vi "Process.vi"(8 "error in":errorcluster, 11 "Instrument":refnum<class "Instrument.lvclass">) -> (0 "error out":errorcluster, 3 "Instrument out":refnum<class "Instrument.lvclass">)   [LabVIEW 2016, in "Instrument.lvclass"]
doc: "---------------------------------------------------------------\nJKI State Machine Objects™\nhttp://jki.net/state-machine-objects/\nCopyright (C) 2005-2015, JKI <info@jki.net>\nALL RIGHTS RESERVED"
uses:
  Instrument.lvclass
  <vilib>/JKI/JKI SMO/SMO/SMO.lvclass
  <vilib>/JKI/JKI SMO/SMO/Typedefs/Parent Call--Enum.ctl
  levylab_util_remote/src/RemoteControl/RemoteControl.lvclass
  levylab_util_remote/src/RemoteControl/Typedefs/PublicEvents--RemoteControl.ProcessCommand.ctl
  levylab_util_remote/src/RemoteControl/Typedefs/PrivateEvents--RemoteControl.CommandResponse.ctl
  C:/Program Files (x86)/National Instruments/LabVIEW 2016/vi.lib/JKI/JKI SMO/SMO/SMO.lvclass
panel:
  out "ProcessCommand.Data":string
  out "ProcessCommand.Command":string
  # "INSTRUMENT"
  # "Receives command from Remote process"
  # "For instructions on how to use the JKI State Machine Objects, examples and video tutorials, visit:\nhttp://jki.net/state-machine-objects/\n\nJKI State Machine Objects™\nhttp://jki.net/state-machine-objects/\nCopyright (C) 2005-2015, JKI <info@jki.net>\nALL RIGHTS RESERVED"
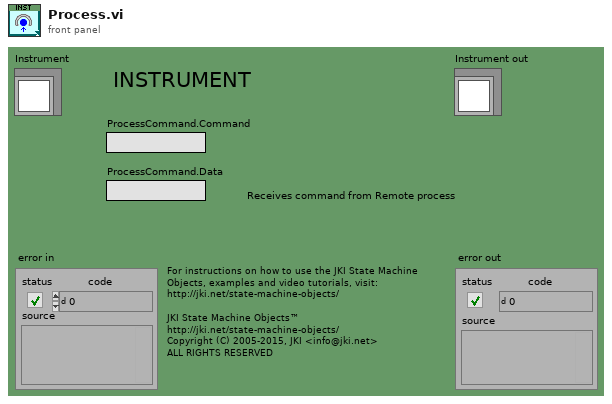
[diagram p1: front panel]
types:
  T1 = typedef "SMO.lvclass/Parent Call--Enum.ctl" = enum16{"Allows parent to run", "Does not request parent to run"}
  T2 = enum32{"invalid app kind", "Development System", "Run Time System", "Student Edition", "Embedded LabVIEW", "Evaluation", "Custom"}
  T3 = enum32{"Invalid", "Standard", "Closed", "Hidden", "Minimized", "Maximized"}
  T4 = enum32{"Bad", "Idle", "Run top level", "Running"}
  T5 = typedef "RemoteControl.lvclass/PrivateEvents--RemoteControl.CommandResponse.ctl" = cluster{"Command Reply":string, "Data Reply":string}
  T6 = typedef "RemoteControl.lvclass/PublicEvents--RemoteControl.ProcessCommand.ctl" = cluster{"Command":string, "Data":string}
  T7 = cluster{"Core":cluster{"Current VI Reference":refnum<vi>, "Close Panel on Exit?":bool, "error":errorcluster}, "Self Reference":refnum<class "Instrument.lvclass">, "Your string data":string, "RemoteControl out":refnum<class "RemoteControl.lvclass">, "ProcessCommand":T6}
  T8 = typedef "Instrument.lvclass/PrivateEvents--Instrument.SetPort.ctl" = i32
  T9 = typedef "Instrument.lvclass/PrivateEvents--Instrument.SetCommands.ctl" = string[]
  T10 = typedef "Instrument.lvclass/PrivateEvents--Instrument.SetAllowedRemote.ctl" = string
  T11 = cluster{"Current VI Reference":refnum<vi>, "Close Panel on Exit?":bool, "error":errorcluster}
  T12 = typedef "SMO.lvclass/Protected Events.ctl" = cluster{"StopProcesses":refnum<user-event>, "AbortProcesses":refnum<user-event>, "Config Changed":refnum<user-event>, "Dependency":refnum<user-event>}
  T13 = typedef "RemoteControl.lvclass/PublicEvents--Cluster.ctl" = cluster{"ProcessCommand":refnum<user-event>}
  T14 = typedef "Instrument.lvclass/PrivateEvents--Cluster.ctl" = cluster{"SetPort":refnum<user-event>, "SetCommands":refnum<user-event>, "SetAllowedRemote":refnum<user-event>}
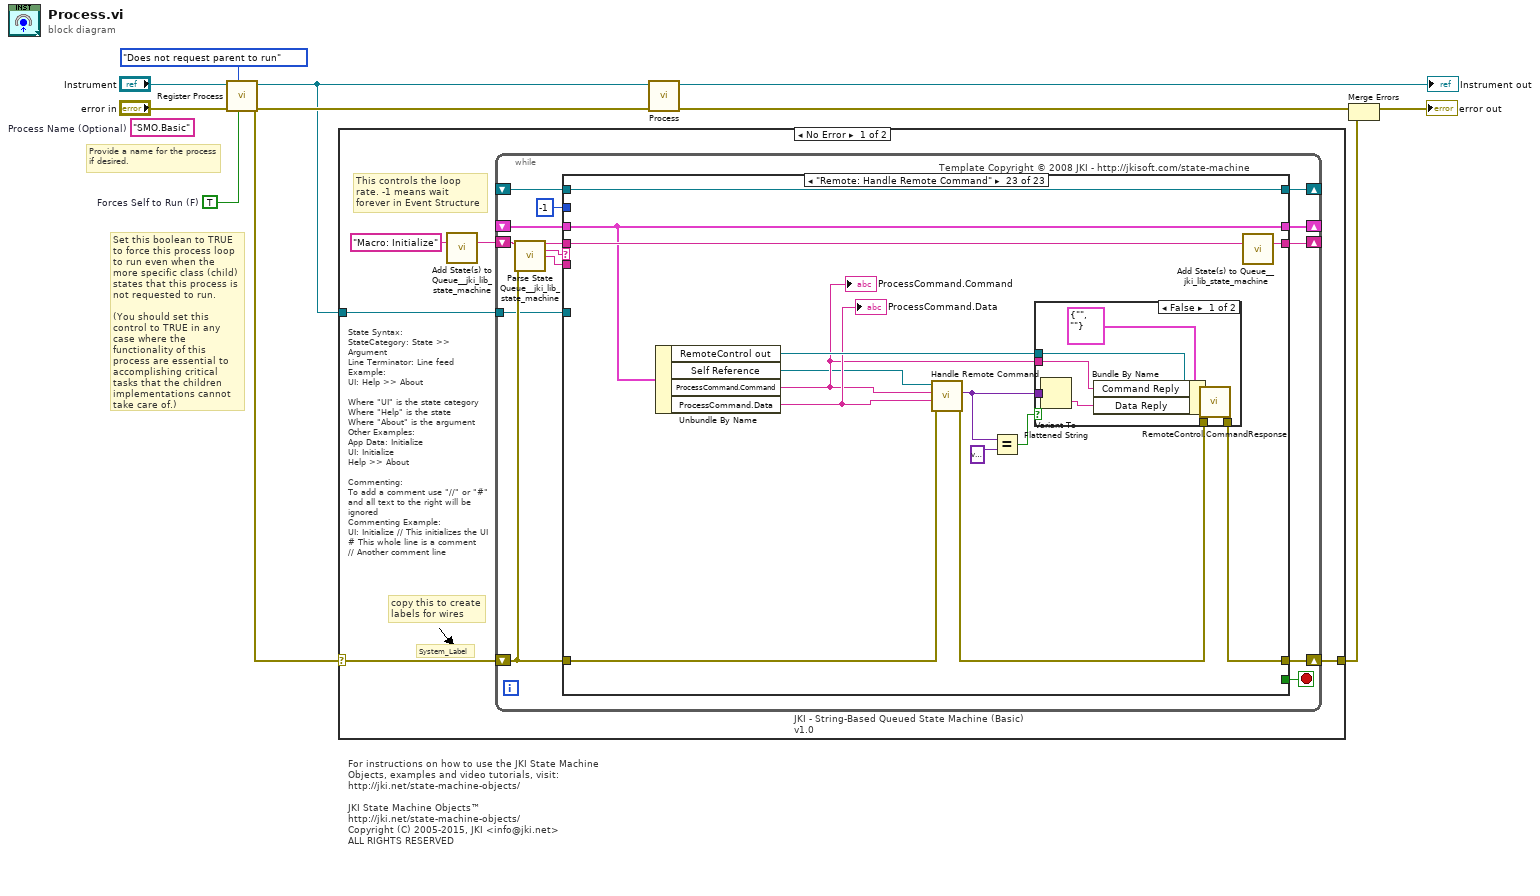
[diagram p0: block diagram]
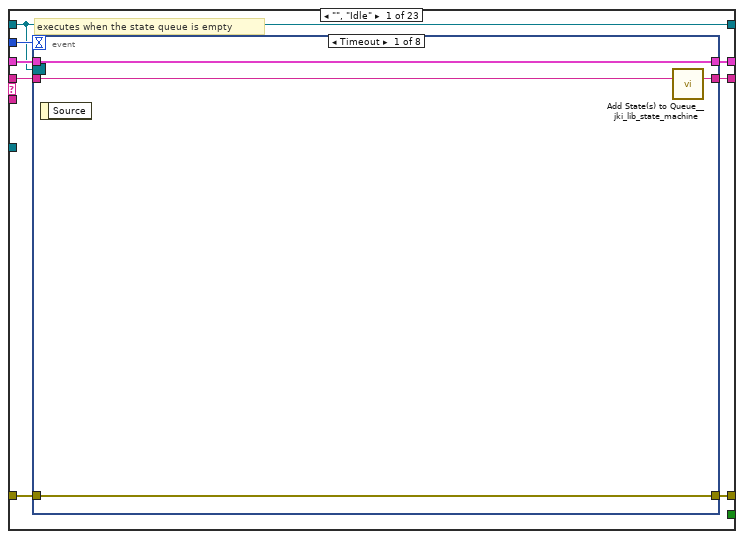
[diagram p2: hidden frame]
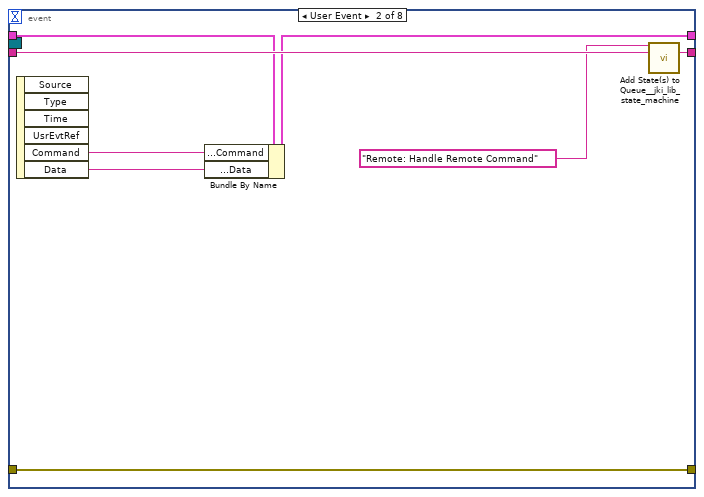
[diagram p3: hidden frame]
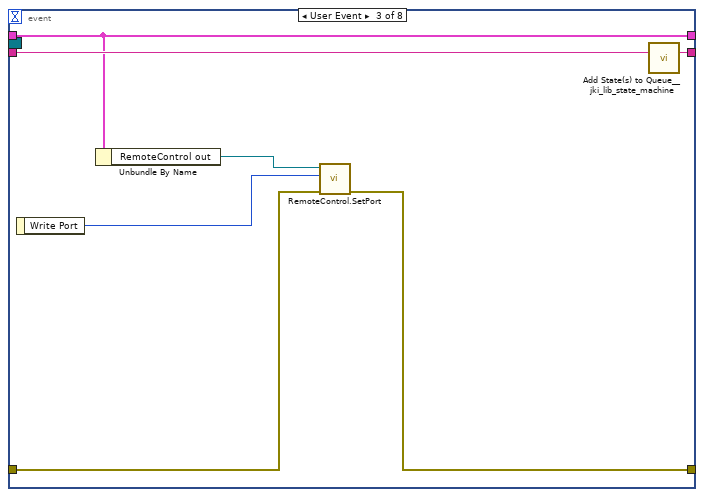
[diagram p4: hidden frame]
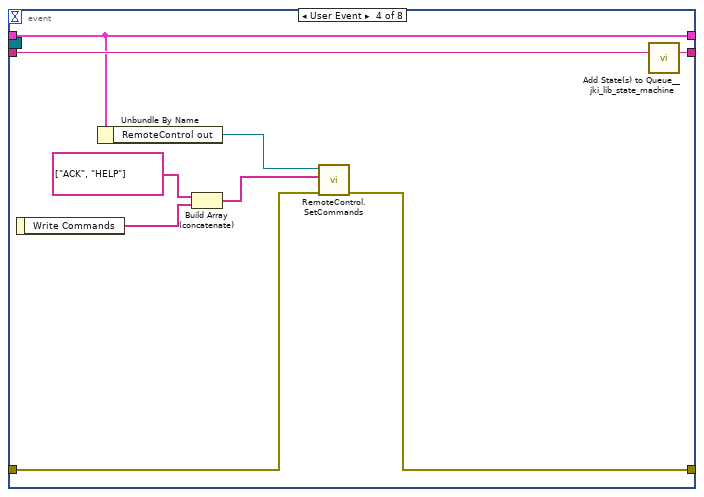
[diagram p5: hidden frame]
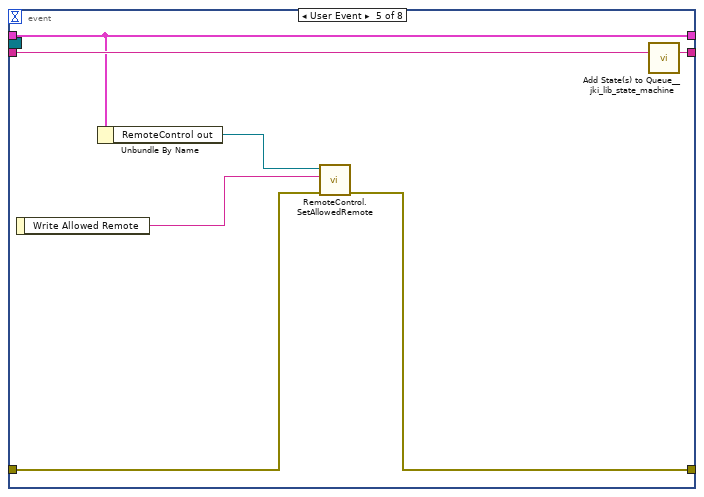
[diagram p6: hidden frame]
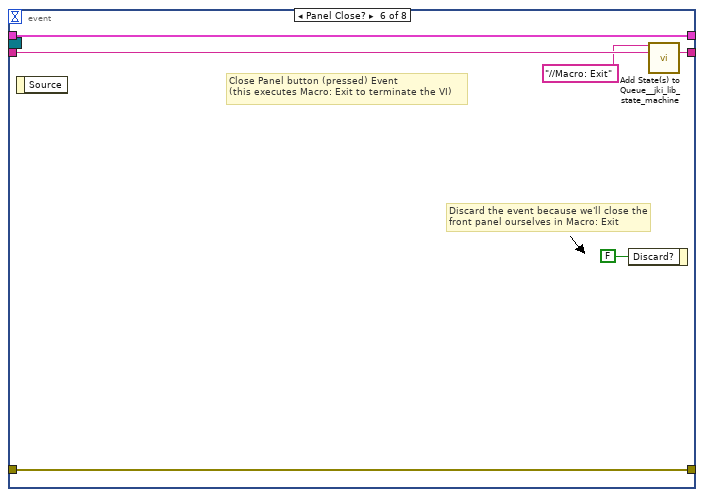
[diagram p7: hidden frame]
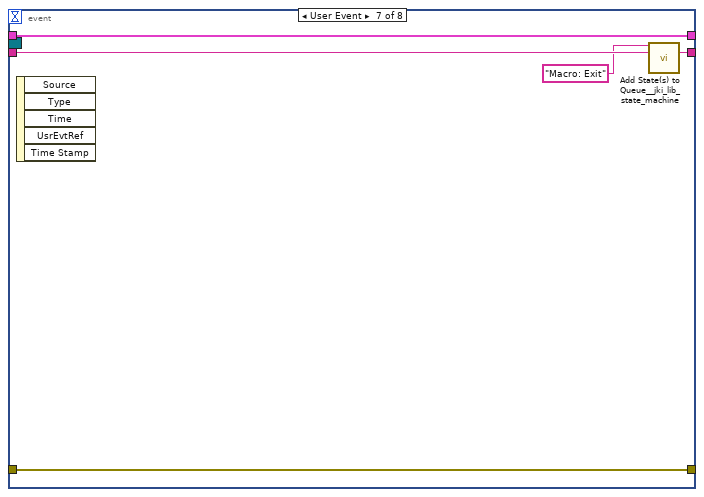
[diagram p8: hidden frame]
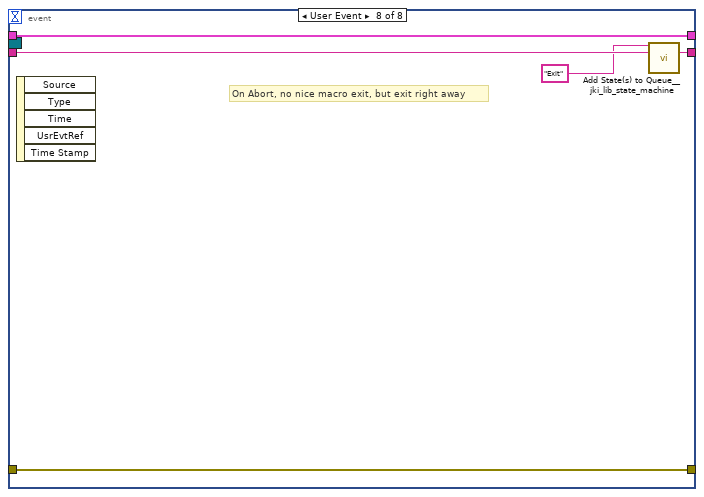
[diagram p9: hidden frame]
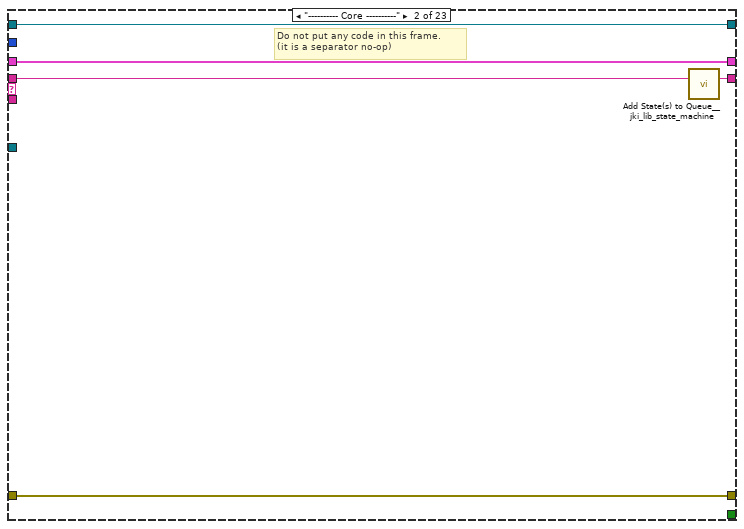
[diagram p10: hidden frame]
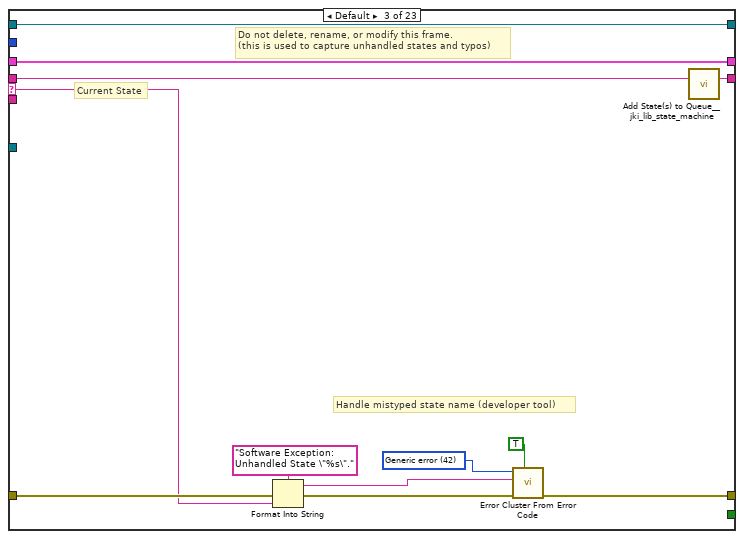
[diagram p11: hidden frame]
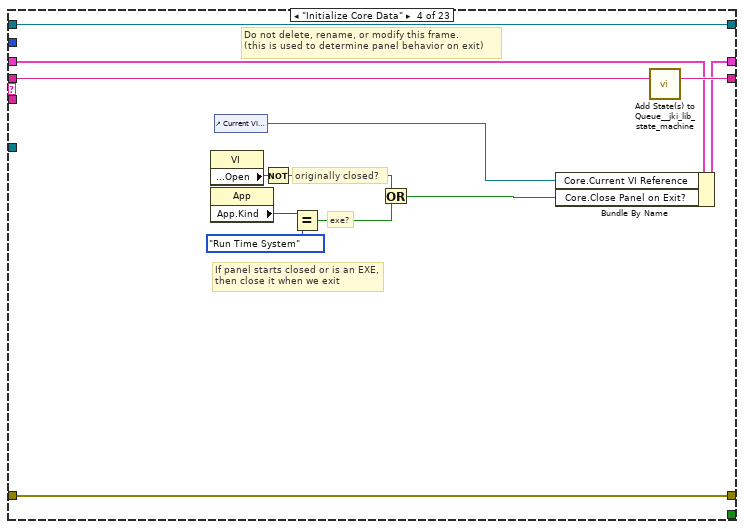
[diagram p12: hidden frame]
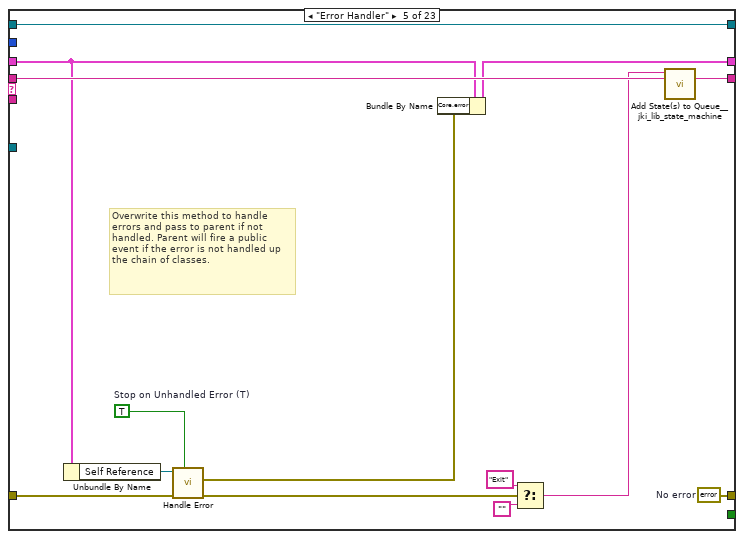
[diagram p13: hidden frame]
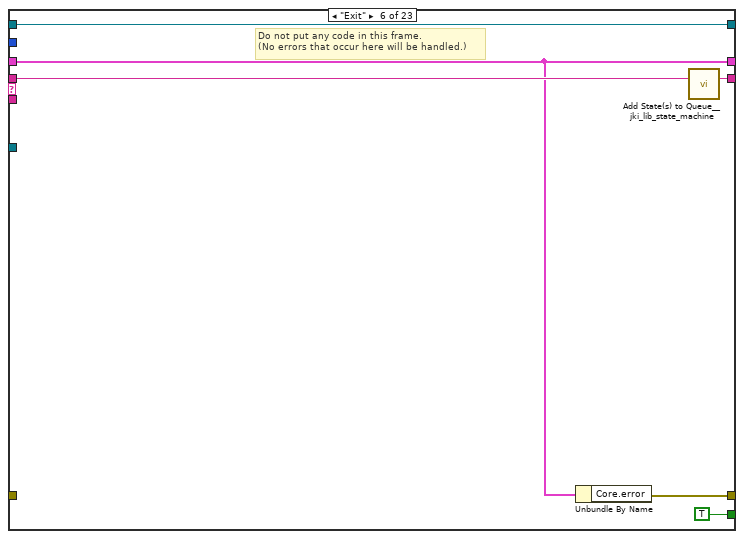
[diagram p14: hidden frame]
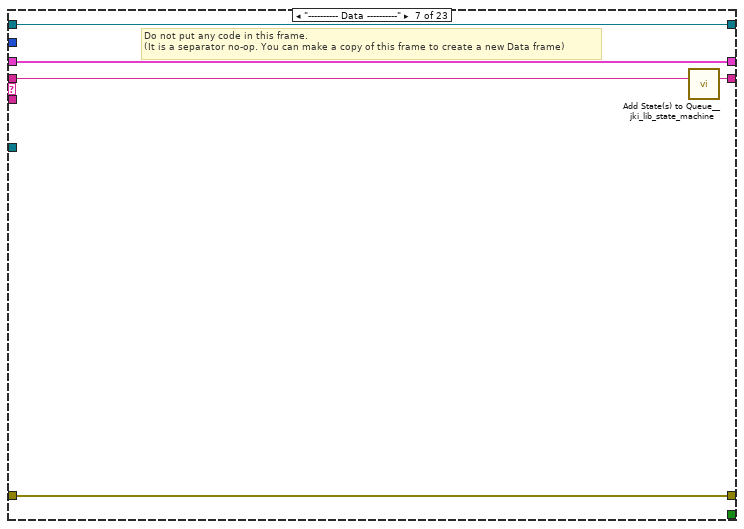
[diagram p15: hidden frame]
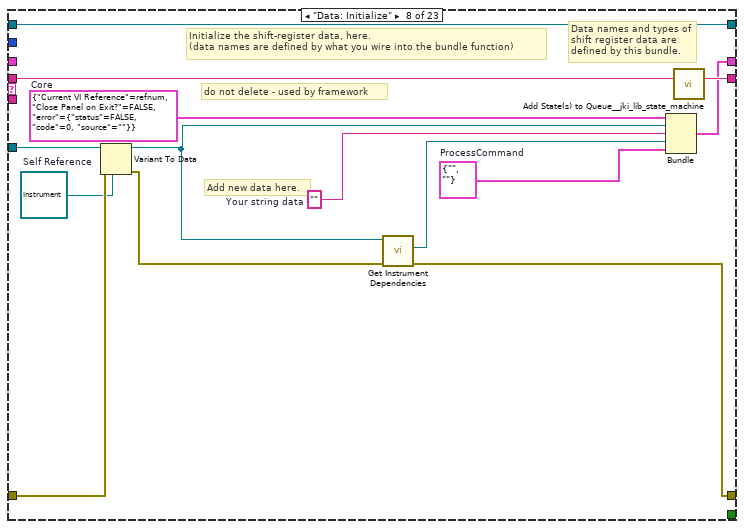
[diagram p16: hidden frame]
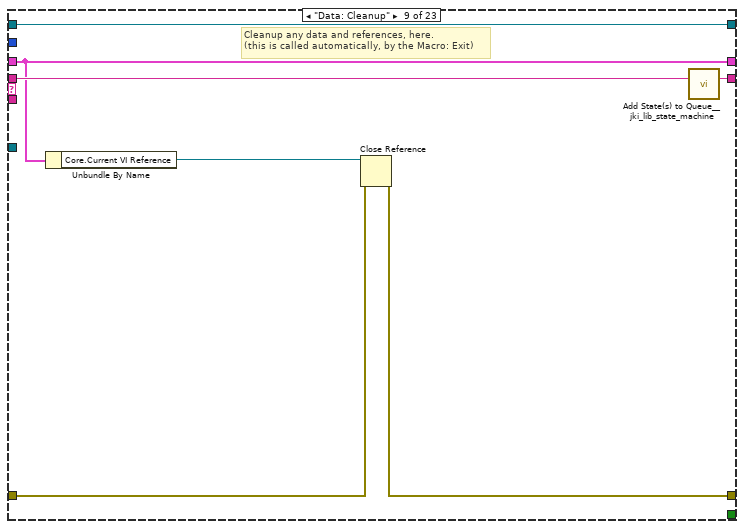
[diagram p17: hidden frame]
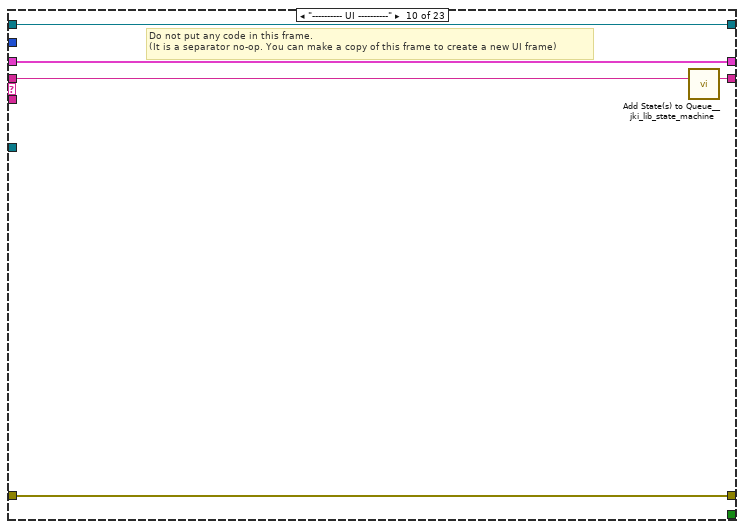
[diagram p18: hidden frame]
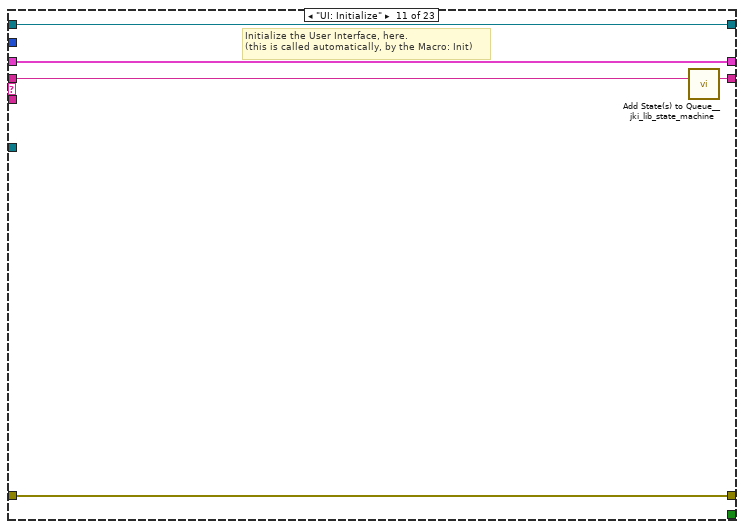
[diagram p19: hidden frame]
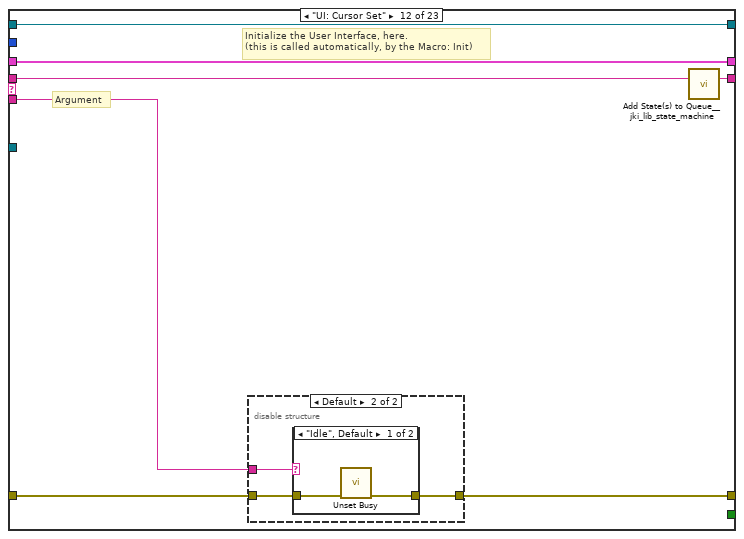
[diagram p20: hidden frame]
diagram:
  w1 = TRUE  # Forces Self to Run (F)
  (unwired) "SMO.Basic"  # Process Name (Optional)
  # "Provide a name for the process\nif desired."
  # "Set this boolean to TRUE to force this process loop to run even when the more specific class (child) states that this process is not requested to run.\n\n(You should set this control to TRUE in any case where the functionality of this process are essential to accomplishing critical tasks that the children implementations cannot take care of.)"
  # "For instructions on how to use the JKI State Machine Objects, examples and video tutorials, visit:\nhttp://jki.net/state-machine-objects/\n\nJKI State Machine Objects™\nhttp://jki.net/state-machine-objects/\nCopyright (C) 2005-2015, JKI <info@jki.net>\nALL RIGHTS RESERVED"
  n1 = call <vilib>:"Register Process.vi"("Forces Self to Run (F)"=w1, "Parent Call"=Parent_Call--Enum."Does not request parent to run", "error in (no error)"="error in", "SMO"="Instrument") -> ("error out"=w7:errorcluster, "SMO out"=w6:refnum<class "Instrument.lvclass">)  [unwired: 6 in]
  n2 = case shown="No Error" w7 {
    selector: w7 -> [w12 w329]
    tunnel: w6 -> [w13 _]
    tunnel: [w11 w329] -> w3
    frame No Error {
      # "State Syntax:\nStateCategory: State >> Argument\nLine Terminator: Line feed\nExample:\nUI: Help >> About\n\nWhere \"UI\" is the state category\nWhere \"Help\" is the state\nWhere \"About\" is the argument\nOther Examples:\nApp Data: Initialize\nUI: Initialize\nHelp >> About\n\nCommenting:\nTo add a comment use \"//\" or \"#\" and all text to the right will be ignored\nCommenting Example:\nUI: Initialize // This initializes the UI\n# This whole line is a comment\n// Another comment line"
      # "copy this to create labels for wires"
      # "This controls the loop rate. -1 means wait forever in Event Structure"
      # "System_Label"
      n3 = call <vilib>:"Add State(s) to Queue__jki_lib_state_machine.vi"("State(s) in (\"\")"="Macro: Initialize") -> ("States Out"=w15:string)  [unwired: 14 in]
      n4 = while "JKI - String-Based Queued State Machine (Basic) v1.0" {
        shift-right: [w22] -> _
        shift-left: _ -> [w21]
        shift-right: [w25] -> w11
        shift-left: w12 -> [w19]
        shift-right: [w24] -> _
        shift-left: w15 -> [w26]
        tunnel: w13 -> [w18]
        shift-right: [w17] -> _
        shift-left: _ -> [w16]
        stop <- w23 stop-if-true
        # "Template Copyright © 2008 JKI - http://jkisoft.com/state-machine"
        n5 = call <vilib>:"Parse State Queue__jki_lib_state_machine.vi"("State Queue"=w26, "Error In (no error)"=w19) -> ("Remaining States"=w28:string, "Current State"=w29:string, "Arguments"=w27:string)  [unwired: 11 in]
        n6 = case shown="\"Remote: Handle Remote Command\"" w29 {
          selector: w29 -> [_ _ w95 _ _ _ _ _ _ _ _ _ _ _ _ _ _ _ _ _ _ _ _]
          tunnel: w28 -> [w37 w93 w99 w118 w132 w138 w143 w157 w164 w169 w174 w181 w197 w229 w243 w257 w262 w273 w278 w294 w300 w305 w319]
          tunnel: w27 -> [_ _ _ _ _ _ _ _ _ _ _ w175 w191 _ _ _ _ _ _ _ _ _ _]
          tunnel: w21 -> [w35 w90 w97 w109 w126 w134 w140 _ w159 w166 w172 w179 w193 w226 w239 w248 w259 w270 w275 w292 w298 w303 w309]
          tunnel: [w34 w91 w101 w115 w127 w133 w141 w146 w160 w167 w171 w176 w194 w227 w241 w255 w260 w264 w276 w288 w296 w301 w310] -> w25
          tunnel: w19 -> [w33 w91 w100 w115 w128 _ w141 w153 w161 w167 w171 w177 w195 w227 w241 w255 w260 w265 w276 w284 w296 w301 w312]
          tunnel: [w36 w92 w98 w117 w131 w137 w142 w156 w163 w168 w173 w180 w196 w228 w242 w256 w261 w272 w277 w293 w299 w304 w318] -> w24
          tunnel: [_ _ _ _ _ TRUE _ _ _ _ _ _ _ _ _ _ _ _ _ _ _ _ _] -> w23
          tunnel: [w32 w90 w97 w116 w125 w134 w140 w155 w159 w166 w172 w179 w193 w226 w239 w248 w259 w270 w275 w292 w298 w303 w309] -> w22
          tunnel: -1 ("Timeout") -> [w31 _ _ _ _ _ _ _ _ _ _ _ _ _ _ _ _ _ _ _ _ _ _]
          tunnel: w18 -> [_ _ _ _ _ _ _ w151 _ _ _ _ _ _ _ _ _ _ _ _ _ _ _]
          tunnel: [w30 w89 w94 w106 w130 w135 w139 w150 w158 w165 w170 w178 w190 w225 w240 w249 w258 w271 w274 w291 w297 w302 w317] -> w17
          tunnel: w16 -> [w30 w89 w94 w106 w130 w135 w139 w150 w158 w165 w170 w178 w190 w225 w240 w249 w258 w271 w274 _ w297 w302 w317]
          frame "", "Idle" {
            # "executes when the state queue is empty"
            n7 = event shown="[0] Timeout" {
              selector: w30 -> [_ _ _ _ _ _ _ _]
              dyn-events: _ -> [_ _ _ _ _ _ _ _]
              timeout: w31 -> [_ _ _ _ _ _ _ _]
              tunnel: w37 -> [w41 w49 w56 w65 w72 w78 w83 w88]
              tunnel: [w40 w48 w55 w64 w71 w77 w82 w87] -> w36
              tunnel: w35 -> [w39 w46 w54 w63 w70 w75 w80 w85]
              tunnel: [w38 w47 w51 w61 w67 w76 w81 w86] -> w34
              tunnel: w33 -> [w38 w47 w52 w62 w68 w76 w81 w86]
              tunnel: [w39 w45 w54 w63 w70 w75 w80 w85] -> w32
              event Timeout {
                n8 = event-data() -> ()  [unwired: 1 in, 1 out]
                n9 = call <vilib>:"Add State(s) to Queue__jki_lib_state_machine.vi"("State(s) in (\"\")"=w41) -> ("States Out"=w40:string)  [unwired: 14 in]
              }
              event User Event {
                n10 = event-data() -> ("Command"=w44:string, "Data"=w43:string)  [unwired: 1 in, 4 out]
                n11 = Bundle By Name(cluster=w46, "ProcessCommand.Command"=w44, "ProcessCommand.Data"=w43) -> (w45:T7)
                n12 = call <vilib>:"Add State(s) to Queue__jki_lib_state_machine.vi"("State(s) in Front (\"\")"="Remote: Handle Remote Command" ("State(s) in Front (\"\")"), "State(s) in (\"\")"=w49) -> ("States Out"=w48:string)  [unwired: 13 in]
              }
              event User Event {
                n13 = event-data() -> ("Write Port"=w53:T8)  [unwired: 1 in]
                n14 = Unbundle By Name(w54) -> ("RemoteControl out"=w50:refnum<class "RemoteControl.lvclass">)
                n15 = call "RemoteControl.SetPort.vi"("error in (no error)"=w52, "Write Port"=w53, "RemoteControl"=w50) -> ("error out"=w51:errorcluster)  [unwired: 7 in, 1 out]
                n16 = call <vilib>:"Add State(s) to Queue__jki_lib_state_machine.vi"("State(s) in (\"\")"=w56) -> ("States Out"=w55:string)  [unwired: 14 in]
              }
              event User Event {
                n17 = event-data() -> ("Write Commands"=w58:T9)  [unwired: 1 in]
                n18 = Unbundle By Name(w63) -> ("RemoteControl out"=w60:refnum<class "RemoteControl.lvclass">)
                n19 = Build Array (concatenate)(string[] ["ACK", "HELP"], w58) -> (w57:T9)
                n20 = call "RemoteControl.SetCommands.vi"("error in (no error)"=w62, "Write Commands"=w57, "RemoteControl"=w60) -> ("error out"=w61:errorcluster)  [unwired: 7 in, 1 out]
                n21 = call <vilib>:"Add State(s) to Queue__jki_lib_state_machine.vi"("State(s) in (\"\")"=w65) -> ("States Out"=w64:string)  [unwired: 14 in]
              }
              event User Event {
                n22 = event-data() -> ("Write Allowed Remote"=w66:T10)  [unwired: 1 in]
                n23 = Unbundle By Name(w70) -> ("RemoteControl out"=w69:refnum<class "RemoteControl.lvclass">)
                n24 = call "RemoteControl.SetAllowedRemote.vi"("error in (no error)"=w68, "SetAllowedRemote"=w66, "RemoteControl"=w69) -> ("error out"=w67:errorcluster)  [unwired: 7 in, 1 out]
                n25 = call <vilib>:"Add State(s) to Queue__jki_lib_state_machine.vi"("State(s) in (\"\")"=w72) -> ("States Out"=w71:string)  [unwired: 14 in]
              }
              event Panel Close? {
                # "Discard the event because we'll close the front panel ourselves in Macro: Exit"
                # "Close Panel button (pressed) Event\n(this executes Macro: Exit to terminate the VI)"
                n26 = event-data() -> ()  [unwired: 1 in, 1 out]
                n27 = event-data("Discard?"=FALSE) -> ()  [unwired: 1 in, 1 out]
                n28 = call <vilib>:"Add State(s) to Queue__jki_lib_state_machine.vi"("State(s) in Front (\"\")"="//Macro: Exit", "State(s) in (\"\")"=w78) -> ("States Out"=w77:string)  [unwired: 13 in]
              }
              event User Event {
                n29 = event-data() -> ()  [unwired: 1 in, 5 out]
                n30 = call <vilib>:"Add State(s) to Queue__jki_lib_state_machine.vi"("State(s) in Front (\"\")"="Macro: Exit", "State(s) in (\"\")"=w83) -> ("States Out"=w82:string)  [unwired: 13 in]
              }
              event User Event {
                # "On Abort, no nice macro exit, but exit right away"
                n31 = event-data() -> ()  [unwired: 1 in, 5 out]
                n32 = call <vilib>:"Add State(s) to Queue__jki_lib_state_machine.vi"("State(s) in Front (\"\")"="Exit", "State(s) in (\"\")"=w88) -> ("States Out"=w87:string)  [unwired: 13 in]
              }
            }
          }
          frame "---------- Core ----------" {
            # "Do not put any code in this frame.\n(it is a separator no-op)"
            n33 = call <vilib>:"Add State(s) to Queue__jki_lib_state_machine.vi"("State(s) in (\"\")"=w93) -> ("States Out"=w92:string)  [unwired: 14 in]
          }
          frame Default {
            w104 = 42 items=["No error", "Argument error", "Memory is full", "Out of zone", "End of file", "File already open", "Generic file I/O error", "File not found", "File permission error", "Disk is full", "Duplicate path", "Too many files open", "System feature not enabled", "Resource file not found", "Cannot add resource", "Resource not found", "Image not found", "Image memory error", "Pen does not exist", "Config type invalid", "Config token not found", "Config parse error", "Config memory error", "Bad external code format", "Bad external code offset", "External code not present", "Null window", "Destroy window error", "Null menu", "Print aborted", "Bad print record", "Print driver error", "Windows error during printing", "Memory error during printing", "Print dialog error", "Generic print error", "Invalid device refnum", "Device not found", "Device parameter error", "Device unit error", "Cannot open device", "Device call aborted", "Generic error", "Cancelled by user", "Object ID too low", "Object ID too high", "Object not in heap", "Unknown heap", "Unknown object (invalid DefProc)", "Unknown object (DefProc not in table)", "Message out of range", "Invalid (null) method", "Unknown message", "Manager call not supported", "Bad address", "Network operation in progress", "Network operation timed out", "Connection is busy", "Network attribute not supported", "Network error", "Address in use", "System out of memory", "Connection aborted", "Connection refused", "Not connected", "Already connected", "Connection closed", "Initialization error (interapplication manager)", "Bad occurrence", "Wait on unbound occurrence handler", "Occurrence queue overflow", "Datalog type conflict", "Unused", "Unrecognized type (interapplication manager)", "Memory corrupt", "Failed to make temporary DLL", "Old CIN version", "Drag socket not found", "Failed to load drop-object", "Failed to register OLE object", "Failed to release OLE object", "Format specifier type mismatch", "Unknown format specifier", "Too few format specifiers", "Too many format specifiers", "Scan failed", "Newer CIN version", "Error converting to variant", "Runtime menu error", "Password tampered", "Variant attribute not found", "Incompatible variant data type", "Event data is not available", "Event Store is not present", "Occurrence is not found", "Event Queue is not created", "Event info is not available", "Refnum passed is NULL", "Error retrieving Class GUID", "Error retrieving CoClass GUID", "Error retrieving TypeLib GUID.", "Bad built application magic bytes.", "Specific driver is different from the specific driver associated with the Logical Name.", "There is no session opened to the class driver.", "Max Error", "MAX - Error with config objects", "MAX - Error loading configuration", "MAX - Group not supported"]
            # "Current State"
            # "Do not delete, rename, or modify this frame.\n(this is used to capture unhandled states and typos)"
            # "Handle mistyped state name (developer tool)"
            n34 = Format Into String(format string="Software Exception: Unhandled State \"%s\"." ("message"), error in=w100, w95) -> (resulting string=w103:string, error out=w102:errorcluster)  [unwired: 1 in]
            n35 = call <vilib>:"Error Cluster From Error Code.vi"("show call chain? (False)"=TRUE, "error in (no error)"=w102, "error message (\"\")"=w103, "error code (0)"=w104) -> ("error out"=w101:errorcluster)  [unwired: 5 in]
            n36 = call <vilib>:"Add State(s) to Queue__jki_lib_state_machine.vi"("State(s) in (\"\")"=w99) -> ("States Out"=w98:string)  [unwired: 14 in]
          }
          frame "Initialize Core Data" {
            # "Do not delete, rename, or modify this frame.\n(this is used to determine panel behavior on exit)"
            # "originally closed?"
            # "exe?"
            # "If panel starts closed or is an EXE, then close it when we exit"
            n37 = property class="VI"() -> ("Front Panel.Open"=w114:bool)  [unwired: 2 in, 2 out]
            n38 = property class="App"() -> ("App.Kind"=w113:T2)  [unwired: 2 in, 2 out]
            n39 = control-ref of="Current VI Reference"() -> (w107:refnum<vi>)
            n40 = Not(x=w114) -> (.not. x?=w111:bool)
            n41 = Equal?(x=w113, y=T2."Run Time System" ("Application:Kind")) -> (x = y?=w110:bool)
            n42 = Or(x=w111, y=w110) -> (x .or. y?=w108:bool)
            n43 = Bundle By Name(cluster=w109, "Core.Current VI Reference"=w107, "Core.Close Panel on Exit?"=w108) -> (w116:T7)
            n44 = call <vilib>:"Add State(s) to Queue__jki_lib_state_machine.vi"("State(s) in (\"\")"=w118) -> ("States Out"=w117:string)  [unwired: 14 in]
          }
          frame "Error Handler" {
            w119 = TRUE  # Stop on Unhandled Error (T)
            w127 = errorcluster {"status"=FALSE, "code"=0, "source"=""}  # No error
            # "Overwrite this method to handle errors and pass to parent if not handled. Parent will fire a public event if the error is not handled up the chain of classes."
            n45 = Unbundle By Name(w126) -> ("Self Reference"=w129:refnum<class "Instrument.lvclass">)
            n46 = call-dynamic "Handle Error.vi"("Stop on Unhandled Error (T)"=w119, "error in"=w128, "SMO"=w129) -> ("handling error"=w120:errorcluster, "Unhandled error"=w123:errorcluster)  [unwired: 6 in, 1 out]
            n47 = Bundle By Name(cluster=w126, "Core.error"=w123) -> (w125:T7)
            n48 = Select(t="Exit", s=w120, f="") -> (s? t:f=w124:string)
            n49 = call <vilib>:"Add State(s) to Queue__jki_lib_state_machine.vi"("State(s) in Front (\"\")"=w124, "State(s) in (\"\")"=w132) -> ("States Out"=w131:string)  [unwired: 13 in]
          }
          frame "Exit" {
            # "Do not put any code in this frame.\n(No errors that occur here will be handled.)"
            n50 = Unbundle By Name(w134) -> ("Core.error"=w133:errorcluster)
            n51 = call <vilib>:"Add State(s) to Queue__jki_lib_state_machine.vi"("State(s) in (\"\")"=w138) -> ("States Out"=w137:string)  [unwired: 14 in]
          }
          frame "---------- Data ----------" {
            # "Do not put any code in this frame.\n(It is a separator no-op. You can make a copy of this frame to create a new Data frame)"
            n52 = call <vilib>:"Add State(s) to Queue__jki_lib_state_machine.vi"("State(s) in (\"\")"=w143) -> ("States Out"=w142:string)  [unwired: 14 in]
          }
          frame "Data: Initialize" {
            w144 = T6 {"Command"="", "Data"=""}  # ProcessCommand
            w149 = T11 {"Current VI Reference"=refnum, "Close Panel on Exit?"=FALSE, "error"={"status"=FALSE, "code"=0, "source"=""}}  # Core
            w152 = refnum<class "Instrument.lvclass"> refnum  # Self Reference
            w154 = ""  # Your string data
            # "do not delete - used by framework"
            # "Add new data here."
            # "Data names and types of shift register data are defined by this bundle."
            # "Initialize the shift-register data, here.\n(data names are defined by what you wire into the bundle function)"
            n53 = Variant To Data(error in=w153, type=w152, Variant=w151) -> (data=w148:refnum<class "Instrument.lvclass">, error out=w145:errorcluster)
            n54 = call "Get Instrument Dependencies.vi"("error in (no error)"=w145, "Instrument in"=w148) -> ("error out"=w146:errorcluster, "RemoteControl out"=w147:refnum<class "RemoteControl.lvclass">)  [unwired: 7 in, 1 out]
            n55 = Bundle("Core"=w149, "Self Reference"=w148, "Your string data"=w154, "RemoteControl out"=w147, "ProcessCommand"=w144) -> (w155:T7)  [unwired: 1 in]
            n56 = call <vilib>:"Add State(s) to Queue__jki_lib_state_machine.vi"("State(s) in (\"\")"=w157) -> ("States Out"=w156:string)  [unwired: 14 in]
          }
          frame "Data: Cleanup" {
            # "Cleanup any data and references, here.\n(this is called automatically, by the Macro: Exit)"
            n57 = Unbundle By Name(w159) -> ("Core.Current VI Reference"=w162:refnum<vi>)
            n58 = Close Reference(reference=w162, error in (no error)=w161) -> (error out=w160:errorcluster)
            n59 = call <vilib>:"Add State(s) to Queue__jki_lib_state_machine.vi"("State(s) in (\"\")"=w164) -> ("States Out"=w163:string)  [unwired: 14 in]
          }
          frame "---------- UI ----------" {
            # "Do not put any code in this frame.\n(It is a separator no-op. You can make a copy of this frame to create a new UI frame)"
            n60 = call <vilib>:"Add State(s) to Queue__jki_lib_state_machine.vi"("State(s) in (\"\")"=w169) -> ("States Out"=w168:string)  [unwired: 14 in]
          }
          frame "UI: Initialize" {
            # "Initialize the User Interface, here.\n(this is called automatically, by the Macro: Init)"
            n61 = call <vilib>:"Add State(s) to Queue__jki_lib_state_machine.vi"("State(s) in (\"\")"=w174) -> ("States Out"=w173:string)  [unwired: 14 in]
          }
          frame "UI: Cursor Set" {
            # "Argument"
            # "Initialize the User Interface, here.\n(this is called automatically, by the Macro: Init)"
            n62 = disable-structure shown="Default" {
              disable-tunnel: w177 -> [w182 w185]
              disable-tunnel: [w182 w184] -> w176
              disable-tunnel: w175 -> [_ w183]
              frame condition #0 {
              }
              frame condition #1 (active) {
                n63 = case shown="\"Idle\", Default" w183 {
                  tunnel: w185 -> [w187 w189]
                  tunnel: [w186 w188] -> w184
                  frame "Idle", Default {
                    n64 = call <vilib>:"Unset Busy.vi"("error in (no error)"=w187) -> ("error out"=w186:errorcluster)  [unwired: 10 in]
                  }
                  frame "Busy" {
                    n65 = call <vilib>:"Set Busy.vi"("error in (no error)"=w189) -> ("error out"=w188:errorcluster)  [unwired: 9 in, 1 out]
                  }
                }
              }
            }
            n66 = call <vilib>:"Add State(s) to Queue__jki_lib_state_machine.vi"("State(s) in (\"\")"=w181) -> ("States Out"=w180:string)  [unwired: 14 in]
          }
          frame "UI: Front Panel State" {
            # "Argument"
            # "Set Front Panel Open or Closed\n(Usage: \"UI: Front Panel State >> Open|Close\")"
            n67 = Unbundle By Name(w193) -> ("Core.Current VI Reference"=w192:refnum<vi>)
            n68 = disable-structure shown="Default" {
              disable-tunnel: w195 -> [w201 w224]
              disable-tunnel: [w200 w224] -> w194
              disable-tunnel: w192 -> [w199 _]
              disable-tunnel: w191 -> [w198 _]
              frame condition #0 (active) {
                n69 = case shown="\"Close\"" w198 {
                  tunnel: w201 -> [w205 w218]
                  tunnel: [w207 w219] -> w200
                  tunnel: w199 -> [w206 w216]
                  frame "Open", Default {
                    n70 = property class="VI"(reference=w206, error in=w205) -> (reference out=w203:refnum<vi>, error out=w204:errorcluster, "FP.State"=w202:T3)
                    n71 = case shown="\"Closed\"" w202 {
                      tunnel: [w210 w213] -> w207
                      tunnel: w204 -> [w209 w213]
                      tunnel: w203 -> [w208 _]
                      frame "Closed" {
                        n72 = invoke class="VI" method="FP.Open"(reference=w208, error in=w209, "Activate"=TRUE, "State"=T3."Standard") -> (error out=w210:errorcluster)  [unwired: 1 in, 4 out]
                      }
                      frame Default {
                      }
                    }
                  }
                  frame "Close" {
                    n73 = property class="VI"(reference=w216, error in=w218) -> (reference out=w215:refnum<vi>, error out=w217:errorcluster, "FP.State"=w214:T3)
                    n74 = case shown="Default" w214 {
                      tunnel: [w220 w223] -> w219
                      tunnel: w217 -> [w220 w222]
                      tunnel: w215 -> [_ w221]
                      frame "Invalid", "Closed" {
                      }
                      frame Default {
                        n75 = invoke class="VI" method="FP.Close"(reference=w221, error in=w222) -> (error out=w223:errorcluster)  [unwired: 1 in, 2 out]
                      }
                    }
                  }
                }
              }
              frame condition #1 {
              }
            }
            n76 = call <vilib>:"Add State(s) to Queue__jki_lib_state_machine.vi"("State(s) in (\"\")"=w197) -> ("States Out"=w196:string)  [unwired: 14 in]
          }
          frame "---------- Macro ----------" {
            # "Do not put any code in this frame.\n(It is a separator no-op. You can make a copy of this frame to create a new Macro frame)"
            n77 = call <vilib>:"Add State(s) to Queue__jki_lib_state_machine.vi"("State(s) in (\"\")"=w229) -> ("States Out"=w228:string)  [unwired: 14 in]
          }
          frame "Macro: Initialize" {
            w234 = "UI: Initialize\nUI: Front Panel State >> Open"  # UI: Initialize UI: Front Panel State >> Open
            w230 = "Process: Sync"
            # "Initialization Macro\n(This is called once, when the VI starts)"
            n78 = control-ref of="This VI"() -> (w232:refnum<vi>)
            n79 = property class="VI"(reference=w232) -> ("Exec.State"=w231:T4)  [unwired: 1 in, 2 out]
            n80 = Equal?(x=w231, y=T4."Run top level") -> (x = y?=w237:bool)
            n81 = Select(t=w230, s=w237, f="") -> ()  [unwired: 1 out]
            n82 = call <vilib>:"Add State(s) to Queue__jki_lib_state_machine.vi"("State(s) in Front (\"\")"="Data: Initialize\nInitialize Core Data\nEvents: Register", "State(s) in (\"\")"=w230, "State(s) at Back (\"\")"=w234) -> ("States Out"=w233:string)  [unwired: 12 in]
            n83 = call <vilib>:"Add State(s) to Queue__jki_lib_state_machine.vi"("State(s) in Front (\"\")"=w233, "State(s) in (\"\")"=w243) -> ("States Out"=w242:string)  [unwired: 13 in]
          }
          frame "Macro: Exit" {
            # "Exit Macro\n(This is called once, when the VI exits)"
            n84 = Unbundle By Name(w248) -> ("Core.Close Panel on Exit?"=w254:bool)
            n85 = Select(t="UI: Front Panel State >> Close", s=w254, f="") -> (s? t:f=w251:string)
            n86 = call <vilib>:"Add State(s) to Queue__jki_lib_state_machine.vi"("State(s) in Front (\"\")"="Data: Cleanup\nEvents: Unregister", "State(s) in (\"\")"="Process: Sync", "State(s) at Back (\"\")"="Exit") -> ("States Out"=w245:string)  [unwired: 12 in]
            n87 = call <vilib>:"Add State(s) to Queue__jki_lib_state_machine.vi"("State(s) in (\"\")"=w251, "State(s) at Back (\"\")"=w245) -> ("States Out"=w250:string)  [unwired: 13 in]
            n88 = call <vilib>:"Add State(s) to Queue__jki_lib_state_machine.vi"("State(s) in Front (\"\")"=w250, "State(s) in (\"\")"=w257) -> ("States Out"=w256:string)  [unwired: 13 in]
          }
          frame "---------- Process ----------" {
            # "Template Separator\n(You can make a copy of, or modify, this frame)"
            n89 = call <vilib>:"Add State(s) to Queue__jki_lib_state_machine.vi"("State(s) in (\"\")"=w262) -> ("States Out"=w261:string)  [unwired: 14 in]
          }
          frame "Process: Sync" {
            n90 = Unbundle By Name(w270) -> ("Self Reference"=w266:refnum<class "Instrument.lvclass">)
            n91 = call <vilib>:"WaitOnProcessSync.vi"("error in (no error)"=w265, "SMO"=w266) -> ("error out"=w264:errorcluster, "Don't run?"=w269:bool)  [unwired: 7 in, 1 out]
            n92 = Select(t="Data: Cleanup\nEvents: Unregister\nExit", s=w269, f="") -> (s? t:f=w263:string)
            n93 = call <vilib>:"Add State(s) to Queue__jki_lib_state_machine.vi"("State(s) in Front (\"\")"=w263, "State(s) in (\"\")"=w273) -> ("States Out"=w272:string)  [unwired: 13 in]
          }
          frame "---------- Events ----------" {
            # "Template Separator\n(You can make a copy of, or modify, this frame)"
            n94 = call <vilib>:"Add State(s) to Queue__jki_lib_state_machine.vi"("State(s) in (\"\")"=w278) -> ("States Out"=w277:string)  [unwired: 14 in]
          }
          frame "Events: Register" {
            # "Expand to add\nmore events"
            n95 = Unbundle By Name(w292) -> ("RemoteControl out"=w283:refnum<class "RemoteControl.lvclass">, "Self Reference"=w289:refnum<class "Instrument.lvclass">)
            n96 = call <vilib>:"GetProtectedEvents.vi"("SMO"=w289) -> ("error out"=w286:errorcluster, "SMO Protected Events"=w290:T12, "SMO out"=w282:refnum<class "Instrument.lvclass">)  [unwired: 8 in]
            n97 = call "RemoteControl.GetPublicEvents.vi"("RemoteControl"=w283) -> ("error out"=w279:errorcluster, "Public Events"=w285:T13)  [unwired: 8 in, 1 out]
            n98 = call "Instrument.GetPrivateEvents.vi"("Instrument"=w282) -> ("error out"=w280:errorcluster, "Private Events"=w281:T14)  [unwired: 8 in, 1 out]
            n99 = register-events(w290, w285, w281) -> (reference out=w291:refnum<event-registration>, error out=w287:errorcluster)  [unwired: 2 in]
            n100 = Merge Errors(w279, w280, w284, w287, w286) -> (w288:errorcluster)
            n101 = call <vilib>:"Add State(s) to Queue__jki_lib_state_machine.vi"("State(s) in (\"\")"=w294) -> ("States Out"=w293:string)  [unwired: 14 in]
          }
          frame "Events: Unregister" {
            n102 = Unregister For Events(event registration refnum=w297, error in=w296) -> (error out=w295:errorcluster)
            n103 = call <vilib>:"Clear Errors.vi"("error in (no error)"=w295) -> ()  [unwired: 5 in, 2 out]
            n104 = call <vilib>:"Add State(s) to Queue__jki_lib_state_machine.vi"("State(s) in (\"\")"=w300) -> ("States Out"=w299:string)  [unwired: 14 in]
          }
          frame "---------- Remote ----------" {
            n105 = call <vilib>:"Add State(s) to Queue__jki_lib_state_machine.vi"("State(s) in (\"\")"=w305) -> ("States Out"=w304:string)  [unwired: 14 in]
          }
          frame "Remote: Handle Remote Command" {
            n106 = Unbundle By Name(w309) -> ("RemoteControl out"=w316:refnum<class "RemoteControl.lvclass">, "Self Reference"=w313:refnum<class "Instrument.lvclass">, "ProcessCommand.Command"=w314:string, "ProcessCommand.Data"=w315:string)
            "ProcessCommand.Command" <- w314
            "ProcessCommand.Data" <- w315
            n107 = call-dynamic "Handle Remote Command.vi"("error in (no error)"=w312, "Data"=w315, "Command"=w314, "Instrument in"=w313) -> ("error out"=w311:errorcluster, "Variant"=w307:variant)  [unwired: 5 in, 1 out]
            n108 = Equal?(x=w307, y=variant) -> (x = y?=w306:bool)
            n109 = case shown="False" w306 {
              tunnel: w316 -> [w327 _]
              tunnel: w314 -> [w323 _]
              tunnel: w311 -> [w322 w328]
              tunnel: [w321 w328] -> w310
              tunnel: w307 -> [w320 _]
              frame False {
                n110 = Variant To Flattened String(Variant=w320) -> (data string=w325:string)  [unwired: 1 out]
                n111 = Bundle By Name(cluster=T5 {"Command Reply"="", "Data Reply"=""} ("CommandResponse"), "Command Reply"=w323, "Data Reply"=w325) -> (w324:T5)
                n112 = call "RemoteControl.CommandResponse.vi"("error in (no error)"=w322, "CommandResponse"=w324, "RemoteControl"=w327) -> ("error out"=w321:errorcluster)  [unwired: 7 in, 1 out]
              }
              frame True {
              }
            }
            n113 = call <vilib>:"Add State(s) to Queue__jki_lib_state_machine.vi"("State(s) in (\"\")"=w319) -> ("States Out"=w318:string)  [unwired: 14 in]
          }
        }
      }
    }
    frame Error {
    }
  }
  n114 = call-parent "Process.vi"("error in"=w7, "SMO"=w6) -> ("error out"=w4:errorcluster, "SMO out"=→"Instrument out":refnum<class "Instrument.lvclass">)  [unwired: 8 in]
  n115 = Merge Errors(w4, w3) -> (→"error out":errorcluster)
